vi "WriteAnalogSettings.vi"(1 "error in (no error)":errorcluster) -> (0 "error out":errorcluster)   [LabVIEW 2009]
uses:
  AnalogSettings.ctt
  <vilib>/Utility/config.llb/NI_LVConfig.lvlib
panel:
  in  "Analog Settings":T1={"PCI 671x Device Number"=1, "Samples per Unit"=10}
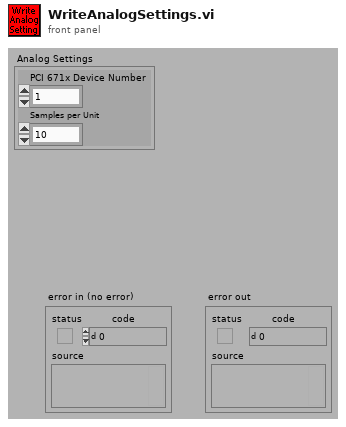
[diagram p1: front panel]
types:
  T1 = typedef "AnalogSettings.ctt" = cluster{"PCI 671x Device Number":u32, "Samples per Unit":u32}
  T2 = typedef "NI_LVConfig.lvlib/Config Data RefNum.ctl" = refnum<k1>
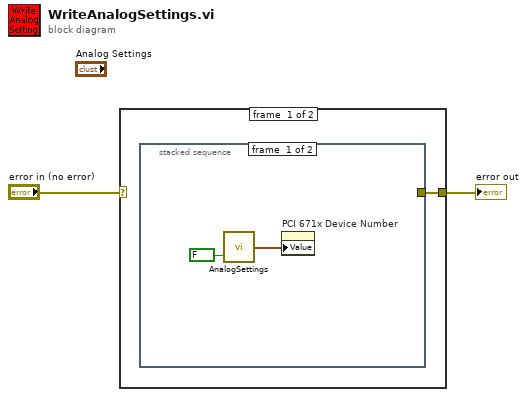
[diagram p0: block diagram]
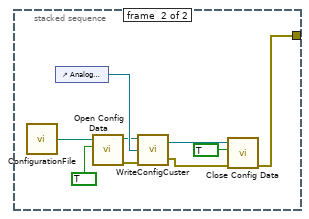
[diagram p2: hidden frame]
diagram:
  n1 = case shown="No Error" "error in (no error)" {
    selector: "error in (no error)" -> [_ w15]
    tunnel: [w3 w15] -> w1
    frame #0 {
      n2 = stacked-sequence {
        tunnel: [_ w11] -> w3
        frame #0 {
          n3 = call "AnalogSettings.vi"("Get/Set"=FALSE) -> ("Analog Settings (output)"=w4:T1)  [unwired: 1 in]
          n4 = property on="PCI 671x Device Number" class="Clust (strict)"("Value"=w4) -> ()  [unwired: 2 in, 2 out]
        }
        frame #1 {
          n5 = call "ConfigurationFile.vi"() -> ("Configuration File (output)"=w9:path)  [unwired: 2 in]
          n6 = control-ref of="Analog Settings"() -> (w10:refnum<vi>)
          n7 = call <vilib>:"Open Config Data.vi"("create file if necessary (T)"=TRUE ("create file if necessary? (T)"), "configuration file path"=w9) -> ("error out"=w6:errorcluster, "refnum"=w7:T2)  [unwired: 7 in, 1 out]
          n8 = call "WriteConfigCuster.vi"("error in (no error)"=w6, "Ctrl Reference"=w10, "ConfigFile (input)"=w7) -> ("error out"=w12:errorcluster, "ConfigFile (output)"=w13:T2)
          n9 = call "Close Config Data.vi"("error in (no error)"=w12, "write configuration file? (T)"=TRUE ("write configuration file? (F)"), "refnum"=w13) -> ("error out"=w11:errorcluster)  [unwired: 8 in]
        }
      }
    }
    frame #1 {
    }
  }
  "error out" <- w1
